vi "Create APU Register Bus - Multi FPGA.vi"(6 "trigger line.<user name>":refnum<k21>="PXI_Trig0", 8 "go.<user name>":bool, 9 "master.<user name>":bool, 11 "shared settings.<user name>":T1 {"start" format="%#.15g"}) -> (0 "go?":bool, 1 "master?":bool, 3 "register bus":T2={"Speed"="Speed", "Crank Angle"="Crank Angle", "Cycle Angle"="Cycle Angle", "Crank Count"="Crank Count", "Cycle Count"="Cycle Count", "1.25 MHz Counter"="1.25 MHz Counter", "Crank Rollover"="Crank Rollover", "Cycle Rollover"="Cycle Rollover", "shared settings"={"start"=0.0, "stuck limit"=0.0}} {"shared settings"."start" format="%#.15g"}, 4 "trigger line":refnum<k21>)   [LabVIEW 2015, in "Engine Simulation Toolkit.lvlib" / "APU.lvlib"]
doc: "Creates the <b>register bus</b> for all components linked to this APU. Place this VI on the root diagram of your FPGA VI and wire the <b>register bus</b> to all components you want sharing speed and position data.\n\nAlso initializes the trigger line to be used for synchronizing multiple FPGAs. Set the <b>trigger line.<user name></b> control to the same value as <b>APU Synchronization Trigger.vi</b> of the same <user name> on all FPGA VIs.\n\nIf this VI will be the timing master, set <b>master.<user name></b> to true."
uses:
  APU.lvlib
  <vilib>/rvi/LocalResourceManager/LocalResourceManager.xnode
  <vilib>/rvi/DataTransferAndStorage/Container/Common/niFpgaContainerGetUniqueNameForEmu.vi
  <vilib>/rvi/DataTransferAndStorage/Container/Common/niFpgaContainerSetEmuInfo.vi
  <vilib>/rvi/eio/common/nirviEmuReportErrorAndStop.vi
  Register Bus.ctl
  Shared Settings.ctl
  <vilib>/eio/EIOMethodNode/EIOMethodNode.xnode
  <vilib>/rvi/eio/common/nirviEmuTemplateMethod_errors.vi
  <vilib>/eio/EIONode/EIONode.xnode
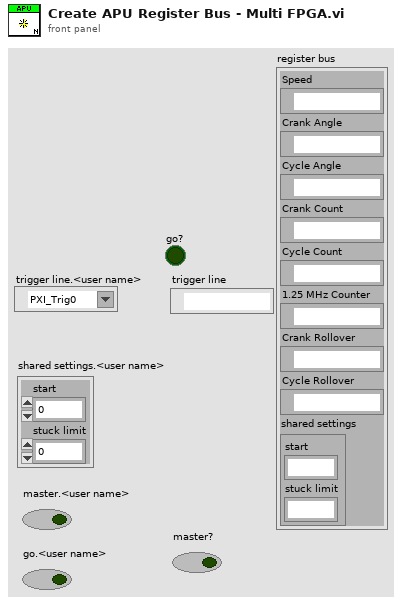
[diagram p1: front panel]
types:
  T1 = typedef "Engine Simulation Toolkit.lvlib/APU.lvlib/Shared Settings.ctl" = cluster{"start":fxp<+,17,17>, "stuck limit":fxp<+,18,18>}
  T2 = typedef "Engine Simulation Toolkit.lvlib/APU.lvlib/Register Bus.ctl" = cluster{"Speed":refnum<k21>, "Crank Angle":refnum<k21>, "Cycle Angle":refnum<k21>, "Crank Count":refnum<k21>, "Cycle Count":refnum<k21>, "1.25 MHz Counter":refnum<k21>, "Crank Rollover":refnum<k21>, "Cycle Rollover":refnum<k21>, "shared settings":T1}
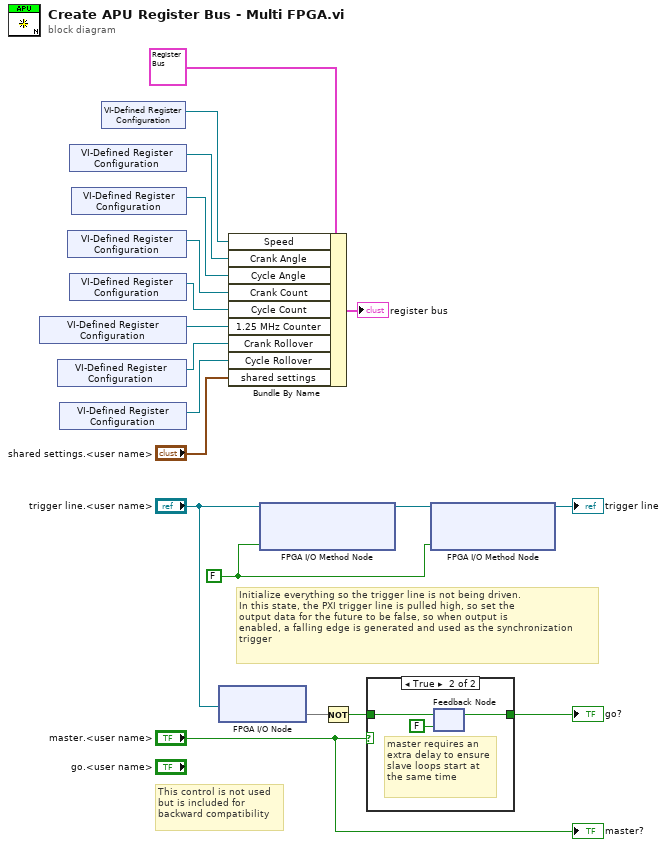
[diagram p0: block diagram]
diagram:
  w7 = FALSE ("Enable")
  # "This control is not used\nbut is included for\nbackward compatibility"
  # "Initialize everything so the trigger line is not being driven.\nIn this state, the PXI trigger line is pulled high, so set the\noutput data for the future to be false, so when output is\nenabled, a falling edge is generated and used as the synchronization\ntrigger"
  n1 = xnode ("VI-Defined Register Configuration")() -> ("Register Out"=w12:refnum<k21>)
  n2 = xnode ("VI-Defined Register Configuration")() -> ("Register Out"=w10:refnum<k21>)
  n3 = xnode ("VI-Defined Register Configuration")() -> ("Register Out"=w9:refnum<k21>)
  n4 = xnode ("VI-Defined Register Configuration")() -> ("Register Out"=w14:refnum<k21>)
  n5 = xnode ("VI-Defined Register Configuration")() -> ("Register Out"=w16:refnum<k21>)
  n6 = xnode ("VI-Defined Register Configuration")() -> ("Register Out"=w13:refnum<k21>)
  n7 = xnode ("VI-Defined Register Configuration")() -> ("Register Out"=w15:refnum<k21>)
  n8 = xnode ("VI-Defined Register Configuration")() -> ("Register Out"=w17:refnum<k21>)
  n9 = xnode "FPGA I/O Node"("FPGA I/O In"="trigger line.<user name>") -> ("I/O Item"=w4)  [unwired: 1 out]
  n10 = Bundle By Name(cluster=T2 {"Speed"="", "Crank Angle"="", "Cycle Angle"="", "Crank Count"="", "Cycle Count"="", "1.25 MHz Counter"="", "Crank Rollover"="", "Cycle Rollover"="", "shared settings"={"start"=0.0, "stuck limit"=0.0}} ("register bus local output v1.0.0"), "Speed"=w17, "Crank Angle"=w16, "Cycle Angle"=w15, "Crank Count"=w14, "Cycle Count"=w13, "1.25 MHz Counter"=w12, "Crank Rollover"=w10, "Cycle Rollover"=w9, "shared settings"="shared settings.<user name>") -> (→"register bus":T2)
  n11 = xnode "FPGA I/O Method Node"("FPGA I/O In"="trigger line.<user name>", "Enable"=w7) -> ("FPGA I/O Out"=w8:refnum<k21>)
  n12 = Not(x=w4) -> (.not. x?=w3:bool)
  n13 = case shown="True" "master.<user name>" {
    tunnel: w3 -> [w20 w23]
    tunnel: [w20 w21] -> w2
    frame False {
    }
    frame True {
      # "master requires an\nextra delay to ensure\nslave loops start at\nthe same time"
      n14 = feedback-in #1(w23) -> ()
      n15 = feedback #1(FALSE) -> (w21:bool)
    }
  }
  "go?" <- w2
  n16 = xnode "FPGA I/O Method Node"("FPGA I/O In"=w8, "Data"=w7) -> ("FPGA I/O Out"=→"trigger line":refnum<k21>)
  "master?" <- "master.<user name>"
